vi "Update IMG Parameter.vi"(0 "connection reference":T1, 1 "K_flat":dbl, 5 "Measuer_ID":i32, 7 "PD":dbl, 9 "WTW":dbl, 11 "error in (no error)":errorcluster caption="错误输入（无错误）", 12 "K_steep":dbl) -> (15 "error out":errorcluster caption="错误输出")   [LabVIEW 2015]
doc: "该模板用于创建子VI。"
uses:
  <vilib>/addons/database/Connection.llb/Conn ObjectReference.ctl
  <vilib>/addons/database/NI_Database_API.lvlib
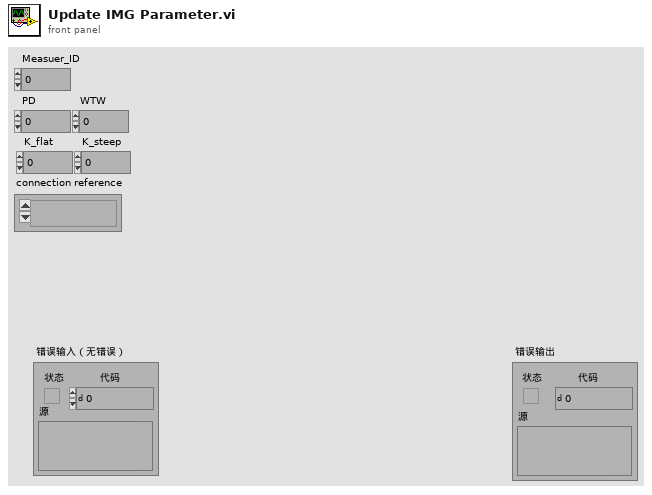
[diagram p1: front panel]
types:
  T1 = typedef "NI_Database_API.lvlib/Conn ObjectReference.ctl" = refnum<k1>
  T2 = cluster{"PD":dbl, "WTW":dbl, "K_flat":dbl, "K_steep":dbl}
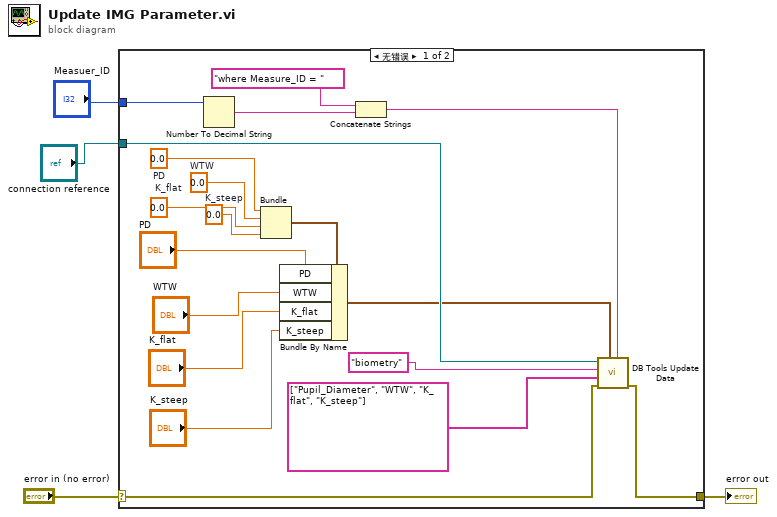
[diagram p0: block diagram]
diagram:
  n1 = case shown="无错误" "error in (no error)" {
    selector: "error in (no error)" -> [w7 w24]
    tunnel: [w6 w24] -> w3
    tunnel: "Measuer_ID" -> [w17 _]
    tunnel: "connection reference" -> [w9 _]
    frame No Error {
      w20 = 0.0  # K_steep
      w21 = 0.0  # K_flat
      w22 = 0.0  # WTW
      w23 = 0.0  # PD
      n2 = Number To Decimal String(number=w17) -> (decimal integer string=w18:string)  [unwired: 1 in]
      n3 = Bundle("PD"=w23, "WTW"=w22, "K_flat"=w21, "K_steep"=w20) -> (w16:T2)  [unwired: 1 in]
      n4 = Bundle By Name(cluster=w16, "PD"="PD", "WTW"="WTW", "K_flat"="K_flat", "K_steep"="K_steep") -> (w8:T2)
      n5 = Concatenate Strings("where Measure_ID = " ("字符串"), w18) -> (w5:string)
      n6 = call <vilib>:"DB Tools Update Data.vi"("condition"=w5, "data"=w8, "error in (no error)"=w7, "columns"=string[] ["Pupil_Diameter", "WTW", "K_flat", "K_steep"], "table"="biometry", "connection reference"=w9) -> ("error out"=w6:errorcluster)  [unwired: 4 in, 1 out]
    }
    frame Error {
    }
  }
  "error out" <- w3
